vi "Abort.vi"(8 "error in (no error)":errorcluster, 11 "NiDaqMx in":refnum<class "NiDaqMx.lvclass">) -> (0 "error out":errorcluster, 3 "NiDaqMx out":refnum<class "NiDaqMx.lvclass">)   [LabVIEW 2018, in "DigitizerPlugins.lvlib" / "NiDaqMx.lvclass"]
uses:
  NiDaqMx.lvclass
  X:/Projects/PMUCal/Modules/Digitizer/DigitizerPlugins/DigitizerBaseClass/DigitizerBase.lvclass
  DigitizerBaseClass/DigitizerBase.lvclass/DigitizerBase.ctl
  NiDaqMx.lvclass/NiDaqMx.ctl
  DigitizerBaseClass/Accessors/Read InstRef.vi
  Accessors/Read TsQue.vi
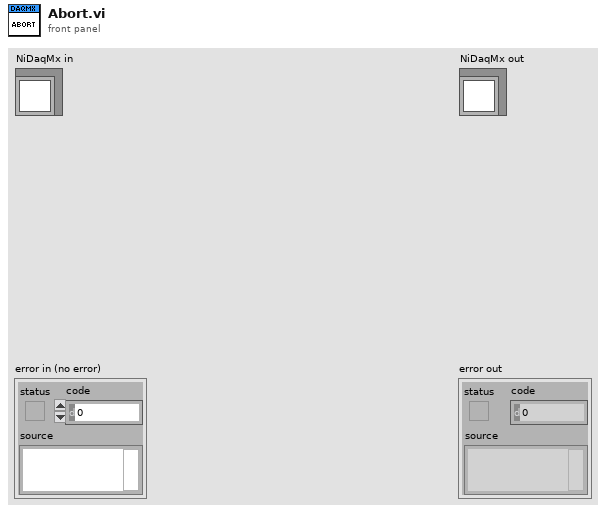
[diagram p1: front panel]
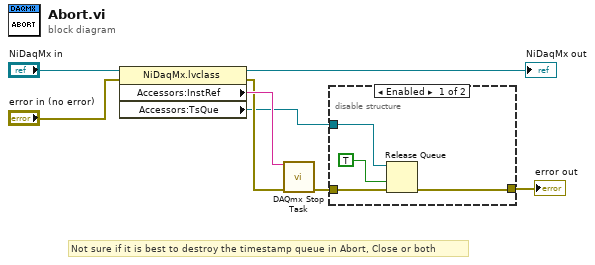
[diagram p0: block diagram]
diagram:
  # "Not sure if it is best to destroy the timestamp queue in Abort, Close or both"
  n1 = property class="NiDaqMx.lvclass"(reference="NiDaqMx in", error in="error in (no error)") -> (reference out=→"NiDaqMx out":refnum<class "NiDaqMx.lvclass">, error out=w6:errorcluster, "Accessors:InstRef"=w7:string, "Accessors:TsQue"=w3:refnum<queue>)
  n2 = call <vilib>:"DAQmx Stop Task.vi"("task/channels in"=w7, "error in"=w6) -> ("error out"=w1:errorcluster)  [unwired: 12 in, 1 out]
  n3 = disable-structure shown="Enabled" {
    disable-tunnel: w3 -> [w11 _]
    disable-tunnel: [w9 w13] -> w2
    disable-tunnel: w1 -> [w12 w13]
    frame Enabled {
      n4 = Release Queue(queue=w11, force destroy? (F)=TRUE, error in (no error)=w12) -> (error out=w9:errorcluster)  [unwired: 2 out]
    }
    frame Disabled {
    }
  }
  "error out" <- w2
